vi "Write Stepper Configuration.vi"(8 "error in (no error)":errorcluster, 10 "Stepper Configuration":T1={"Start"=-0.001, "End"=0.001, "Step"=0.0001, "Append measurements"=[]} {"Step" format="%#_6p"; "End" format="%#_6p"; "Start" format="%#_6p"}, 11 "Stepper in":refnum<class "Stepper.lvclass">) -> (0 "error out":errorcluster, 3 "Stepper out":refnum<class "Stepper.lvclass">)   [LabVIEW 2021, in "Stepper.lvclass"]
uses:
  Stepper.lvclass
  Stepper.lvclass/Stepper.ctl
  NHMFL_Core/Libraries/Instruments/Controls/Stepper Config.ctl
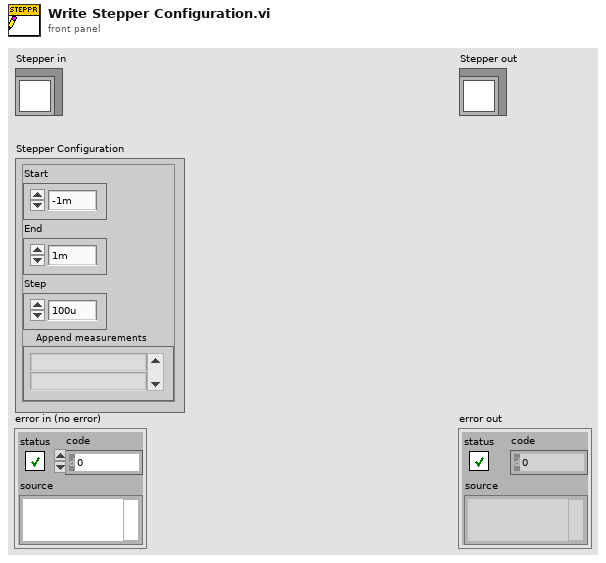
[diagram p1: front panel]
types:
  T1 = typedef "Stepper Config.ctl" = cluster{"Start":dbl, "End":dbl, "Step":dbl, "Append measurements":string[]}
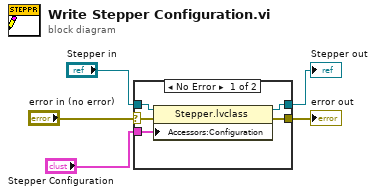
[diagram p0: block diagram]
diagram:
  n1 = case shown="No Error" "error in (no error)" {
    selector: "error in (no error)" -> [w10 w11]
    tunnel: [w9 w11] -> w4
    tunnel: [w7 w12] -> w2
    tunnel: "Stepper in" -> [w8 w12]
    tunnel: "Stepper Configuration" -> [w6 _]
    frame No Error {
      n2 = property class="Stepper.lvclass"(reference=w8, error in=w10, "Accessors:Configuration"=w6) -> (reference out=w7:refnum<class "Stepper.lvclass">, error out=w9:errorcluster)
    }
    frame Error {
    }
  }
  "error out" <- w4
  "Stepper out" <- w2
